vi "sub vi - AI USB4704 (3) v70.vi"() -> (1 "Graph 1":waveform(dbl)[](graph), 2 "Graph 2":waveform(dbl)[](graph), 3 "Graph 3":waveform(dbl)[](graph), 10 "loop time":dbl format="%.6g", 15 "error array":errorcluster[](array[cluster]))   [LabVIEW 2013]
uses:
  program files/Global 1.vi
  <userlib>/DAQNavi Polymorphic VI/create/DAQNavi Create Channel(AI-Voltage).vi
  <userlib>/DAQNavi Polymorphic VI/configure/timing/DAQNavi Timing(Convert Clock).vi
  <userlib>/DAQNavi Polymorphic VI/read/DAQNavi Read (Analog 1D Wfm NChan NSamp).vi
panel:
  in  "SAMPLES":dbl
  in  "RATE(Hz)":dbl
  in  "Tab Control":enum32{"USB #0", "USB #1", "USB #2"}(tab)
  out "physical channels 0":string="DemoDevice,BID#0/ai0:1" caption="property value"
  out "value range 0":string="+/- 5 V" caption="property value"
  out "physical channels 1":string="DemoDevice,BID#0/ai0:1" caption="property value"
  out "value range 1":string="+/- 5 V" caption="property value"
  out "physical channels 2":string="DemoDevice,BID#0/ai0:1" caption="property value"
  out "value range 2":string="+/- 5 V" caption="property value"
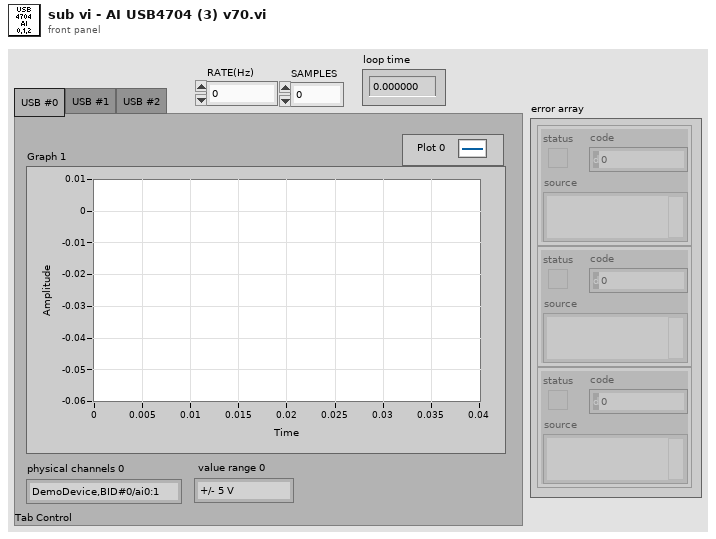
[diagram p1: front panel]
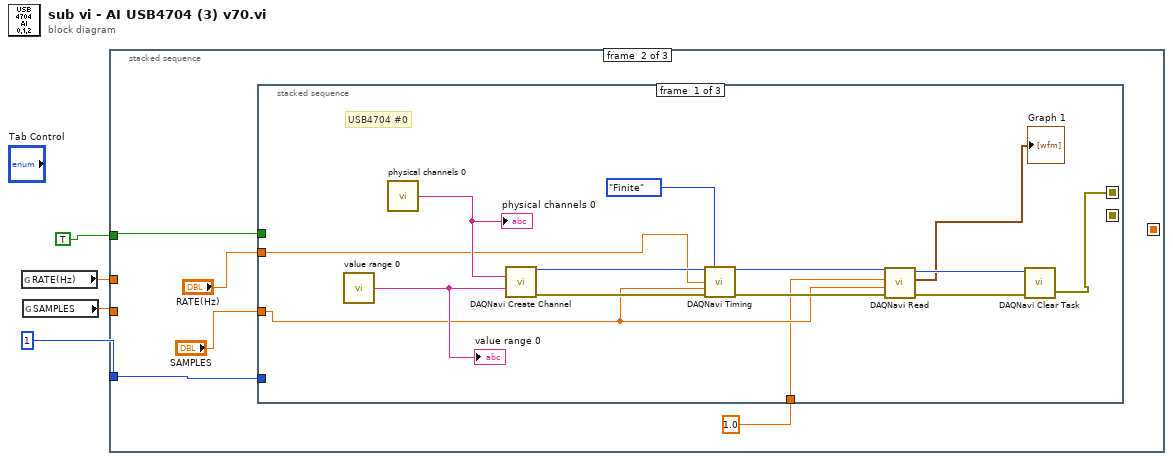
[diagram p0: block diagram]
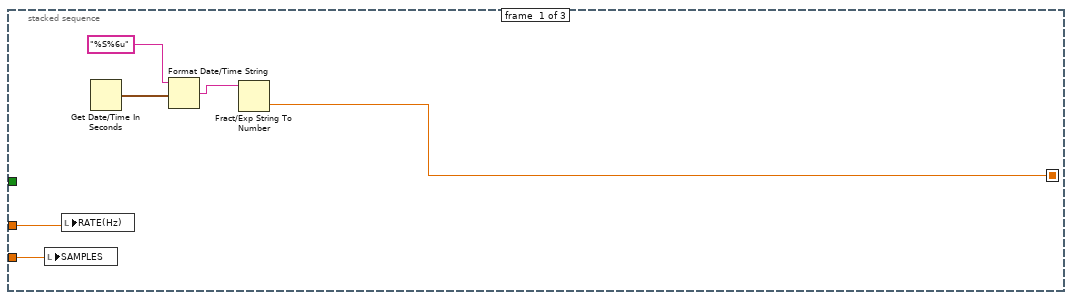
[diagram p2: hidden frame]
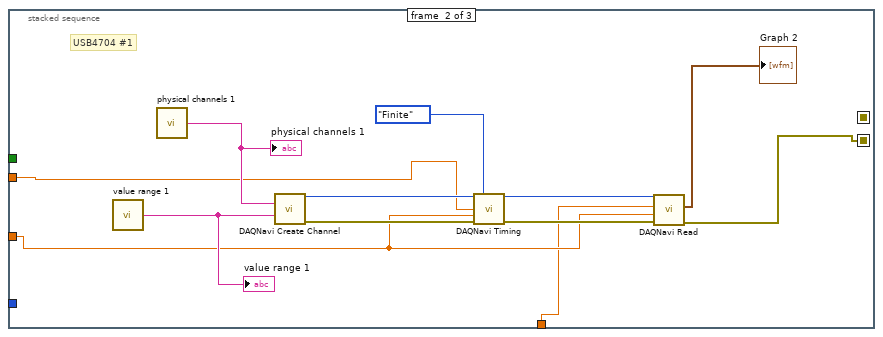
[diagram p3: hidden frame]
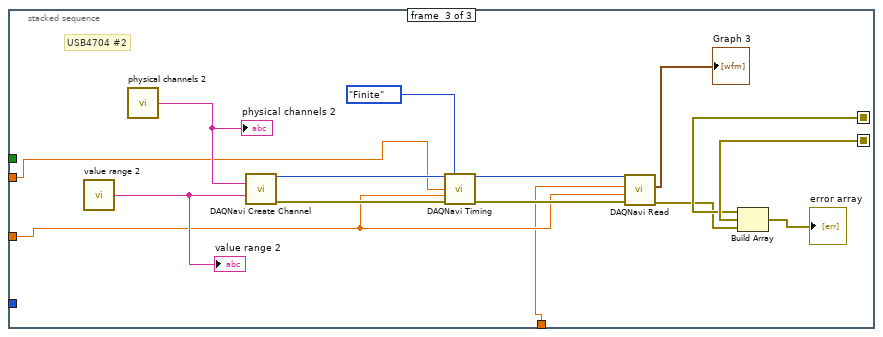
[diagram p4: hidden frame]
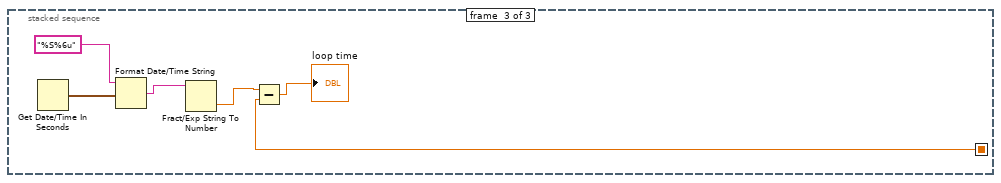
[diagram p5: hidden frame]
diagram:
  n1 = global read "Global 1.vi" "RATE(Hz)"() -> (w3:dbl)
  n2 = global read "Global 1.vi" "SAMPLES"() -> (w2:dbl)
  n3 = stacked-sequence {
    seq-local: [w7 _ _] -> [_ _ w58]
    tunnel: TRUE -> [_ w15 _]
    tunnel: 1 -> [_ w14 _]
    tunnel: w2 -> [w5 _ _]
    tunnel: w3 -> [w6 _ _]
    frame #0 {
      n4 = local write "SAMPLES"(w5) -> ()
      n5 = local write "RATE(Hz)"(w6) -> ()
      n6 = Get Date/Time In Seconds() -> (seconds since 1Jan1904=w9:timestamp)
      n7 = Format Date/Time String(time format string (%c)="%S%6u", seconds (now)=w9) -> (date/time string=w8:string)  [unwired: 1 in]
      n8 = Fract/Exp String To Number(string=w8) -> (number=w7:dbl)  [unwired: 3 in, 1 out]
    }
    frame #1 {
      n9 = stacked-sequence {
        seq-local: [w20 _ _] -> [_ _ w54]
        seq-local: [_ w31 _] -> [_ _ w55]
        tunnel: w15 -> [_ _ _]
        tunnel: "RATE(Hz)" -> [w17 w34 w46]
        tunnel: "SAMPLES" -> [w18 w33 w45]
        tunnel: w14 -> [_ _ _]
        tunnel: 1.0 -> [w16 w30 w42]
        frame #0 {
          # "USB4704 #0"
          n10 = call "value range 0"() -> ("property value"=w21:string)  [unwired: 1 out]
          "value range 0" <- w21
          n11 = call "physical channels 0"() -> ("property value"=w22:string)  [unwired: 1 out]
          "physical channels 0" <- w22
          n12 = call-poly <userlib>:"DAQNavi Create Channel.vi"("physical channels"=w22, "value range"=w21) -> ("task out"=w27:i32, "error out"=w26:errorcluster)  [unwired: 3 in, 9 out]
          n13 = call-poly <userlib>:"DAQNavi Timing.vi"("task in"=w27, "sample mode"=enum16{"Finite", "Continuous"}."Finite", "rate"=w17, "samples per channel"=w18, "error in (no error)"=w26) -> ("task out"=w25:i32, "error out"=w24:errorcluster)  [unwired: 1 in, 8 out]
          n14 = call-poly <userlib>:"DAQNavi Read.vi"("error in (no error)"=w24, "number of samples per channel to read"=w18, "timeout"=w16, "task in"=w25) -> ("error out"=w28:errorcluster, "data"=→"Graph 1":waveform(dbl)[], "task out"=w29:i32)  [unwired: 5 out]
          n15 = call <userlib>:"DAQNavi Clear Task.vi"("error in (no error)"=w28, "task in"=w29) -> ("error out"=w20:errorcluster)  [unwired: 1 out]
        }
        frame #1 {
          # "USB4704 #1"
          n16 = call "value range 1"() -> ("property value"=w35:string)  [unwired: 1 out]
          "value range 1" <- w35
          n17 = call "physical channels 1"() -> ("property value"=w36:string)  [unwired: 1 out]
          "physical channels 1" <- w36
          n18 = call-poly <userlib>:"DAQNavi Create Channel.vi"("physical channels"=w36, "value range"=w35) -> ("task out"=w41:i32, "error out"=w40:errorcluster)  [unwired: 3 in, 9 out]
          n19 = call-poly <userlib>:"DAQNavi Timing.vi"("task in"=w41, "sample mode"=enum16{"Finite", "Continuous"}."Finite", "rate"=w34, "samples per channel"=w33, "error in (no error)"=w40) -> ("task out"=w39:i32, "error out"=w38:errorcluster)  [unwired: 1 in, 8 out]
          n20 = call-poly <userlib>:"DAQNavi Read.vi"("error in (no error)"=w38, "number of samples per channel to read"=w33, "timeout"=w30, "task in"=w39) -> ("error out"=w31:errorcluster, "data"=→"Graph 2":waveform(dbl)[])  [unwired: 6 out]
        }
        frame #2 {
          # "USB4704 #2"
          n21 = call "value range 2"() -> ("property value"=w47:string)  [unwired: 1 out]
          "value range 2" <- w47
          n22 = call "physical channels 2"() -> ("property value"=w48:string)  [unwired: 1 out]
          "physical channels 2" <- w48
          n23 = call-poly <userlib>:"DAQNavi Create Channel.vi"("physical channels"=w48, "value range"=w47) -> ("task out"=w53:i32, "error out"=w52:errorcluster)  [unwired: 3 in, 9 out]
          n24 = call-poly <userlib>:"DAQNavi Timing.vi"("task in"=w53, "sample mode"=enum16{"Finite", "Continuous"}."Finite", "rate"=w46, "samples per channel"=w45, "error in (no error)"=w52) -> ("task out"=w51:i32, "error out"=w50:errorcluster)  [unwired: 1 in, 8 out]
          n25 = call-poly <userlib>:"DAQNavi Read.vi"("error in (no error)"=w50, "number of samples per channel to read"=w45, "timeout"=w42, "task in"=w51) -> ("error out"=w44:errorcluster, "data"=→"Graph 3":waveform(dbl)[])  [unwired: 6 out]
          n26 = Build Array(w54, w55, w44) -> (→"error array":errorcluster[])
        }
      }
    }
    frame #2 {
      n27 = Get Date/Time In Seconds() -> (seconds since 1Jan1904=w61:timestamp)
      n28 = Format Date/Time String(time format string (%c)="%S%6u", seconds (now)=w61) -> (date/time string=w60:string)  [unwired: 1 in]
      n29 = Fract/Exp String To Number(string=w60) -> (number=w59:dbl)  [unwired: 3 in, 1 out]
      n30 = Subtract(x=w59, y=w58) -> (x-y=→"loop time":dbl)
    }
  }
